vi "test-swerve-drive-kinematics-02.vi"() -> (3 "Test Passed":bool)   [LabVIEW 2019]
uses:
  <vilib>/Rock Robotics/WPI/ThirdParty/JAS_Junk/TrajLib/Trajectory_Library.lvlib
  <vilib>/Rock Robotics/WPI/ThirdParty/JAS_Junk/TrajLib/TypeDef/CHASSIS_SPEEDS.ctl
  <vilib>/Rock Robotics/WPI/ThirdParty/JAS_Junk/TrajLib/TypeDef/ROTATION2D.ctl
  <vilib>/Rock Robotics/WPI/ThirdParty/JAS_Junk/TrajLib/TypeDef/SWERVE_DRIVE_MODULE_STATE.ctl
  <vilib>/Analysis/Matrix/Datatypes/RealMatrix.ctl
  <vilib>/Analysis/Matrix/NI_Matrix.lvlib
  <vilib>/Rock Robotics/WPI/ThirdParty/JAS_Junk/TrajLib/TypeDef/TRANSLATION2D.ctl
  <vilib>/Rock Robotics/WPI/ThirdParty/JAS_Junk/TrajLib/TypeDef/SWERVE_DRIVE_KINEMATICS.ctl
panel:
  out "SWERVE_DRIVE_KINEMATICS":T1 {"SavedModuleStates"."Angle"."SIN" format="%13.4f"; "SavedModuleStates"."Angle"."COS" format="%13.4f"; "SavedModuleStates"."Angle"."VALUE" format="%13.4f"; "PrevCoR"."Y" format="%14.3f"; "PrevCoR"."X" format="%14.3f"; "Modules"."Y" format="%14.3f"; "Modules"."X" format="%14.3f"}
  out "module state":T4={"Speed"=0.0, "Angle"={"VALUE"=0.0, "COS"=1.0, "SIN"=0.0}} {"Angle"."SIN" format="%13.4f"; "Angle"."COS" format="%13.4f"; "Angle"."VALUE" format="%13.4f"}
  out "Chassis Speed":T6 {"vOmega" format="%10.3f"; "vY" format="%10.3f"; "vX" format="%10.3f"}
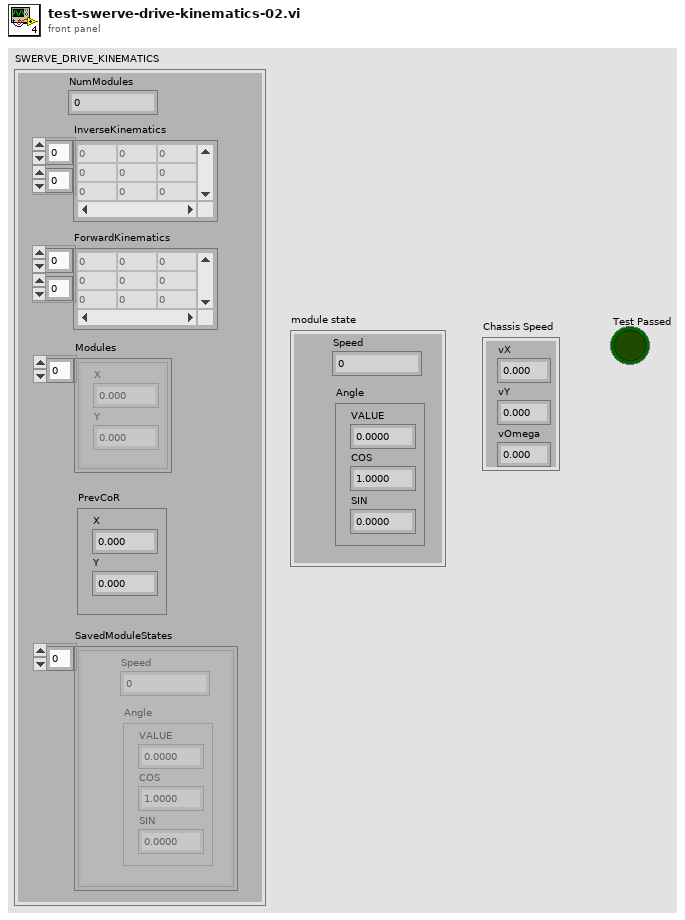
[diagram p1: front panel]
types:
  T1 = typedef "Trajectory_Library.lvlib/SWERVE_DRIVE_KINEMATICS.ctl" = cluster{"NumModules":i32, "InverseKinematics":T2, "ForwardKinematics":T2, "Modules":T3[], "PrevCoR":T3, "SavedModuleStates":T4[]}
  T2 = typedef "NI_Matrix.lvlib/RealMatrix.ctl" = dbl[][]
  T3 = typedef "Trajectory_Library.lvlib/TRANSLATION2D.ctl" = cluster{"X":dbl, "Y":dbl}
  T4 = typedef "Trajectory_Library.lvlib/SWERVE_DRIVE_MODULE_STATE.ctl" = cluster{"Speed":dbl, "Angle":T5}
  T5 = typedef "Trajectory_Library.lvlib/ROTATION2D.ctl" = cluster{"VALUE":dbl, "COS":dbl, "SIN":dbl}
  T6 = typedef "Trajectory_Library.lvlib/CHASSIS_SPEEDS.ctl" = cluster{"vX":dbl, "vY":dbl, "vOmega":dbl}
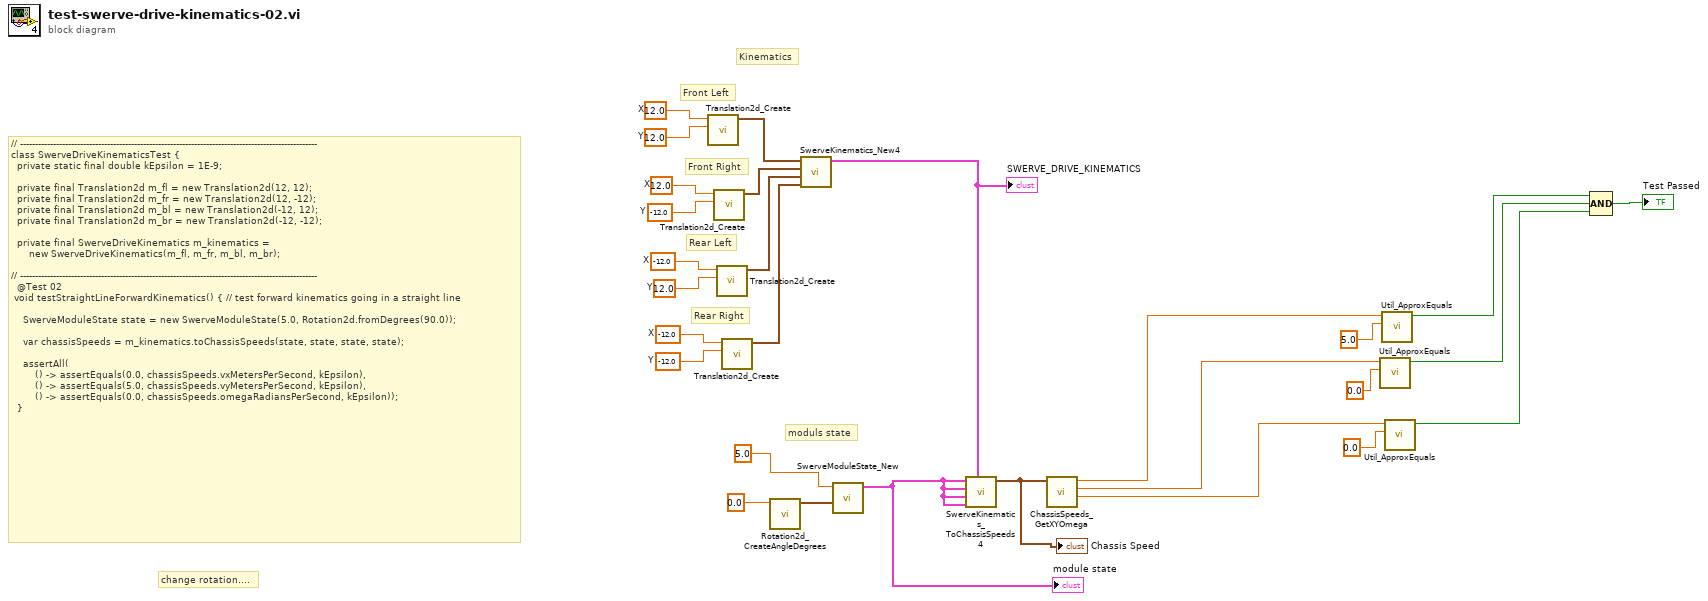
[diagram p0: block diagram]
diagram:
  w24 = -12.0  # X
  w23 = -12.0  # Y
  w22 = -12.0  # X
  w21 = 12.0  # Y
  w20 = 12.0  # X
  w19 = -12.0  # Y
  w18 = 12.0  # X
  w17 = 12.0  # Y
  # "change rotation...."
  # "Kinematics"
  # "Rear Right"
  # "Rear Left"
  # "Front Right"
  # "Front Left"
  # "moduls state"
  # "// ---------------------------------------------------------------------------------------------------\nclass SwerveDriveKinematicsTest {\n  private static final double kEpsilon = 1E-9;\n\n  private final Translation2d m_fl = new Translation2d(12, 12);\n  private final Translation2d m_fr = new Translation2d(12, -12);\n  private final Translation2d m_bl = new Translation2d(-12, 12);\n  private final Translation2d m_br = new Translation2d(-12, -12);\n\n  private final SwerveDriveKinematics m_kinematics =\n      new SwerveDriveKinematics(m_fl, m_fr, m_bl, m_br);\n\n// ---------------------------------------------------------------------------------------------------\n  @Test 02\n void testStraightLineForwardKinematics() { // test forward kinematics going in a straight line\n\n    SwerveModuleState state = new SwerveModuleState(5.0, Rotation2d.fromDegrees(90.0));\n\n    var chassisSpeeds = m_kinematics.toChassisSpeeds(state, state, state, state);\n\n    assertAll(\n        () -> assertEquals(0.0, chassisSpeeds.vxMetersPerSecond, kEpsilon),\n        () -> assertEquals(5.0, chassisSpeeds.vyMetersPerSecond, kEpsilon),\n        () -> assertEquals(0.0, chassisSpeeds.omegaRadiansPerSecond, kEpsilon));\n  }"
  n1 = call <vilib>:"Translation2d_Create.vi"("Y"=w17, "X"=w18) -> ("TRANSLATION"=w25:T3)  [unwired: 9 in]
  n2 = call <vilib>:"Translation2d_Create.vi"("Y"=w19, "X"=w20) -> ("TRANSLATION"=w26:T3)  [unwired: 9 in]
  n3 = call <vilib>:"Translation2d_Create.vi"("Y"=w21, "X"=w22) -> ("TRANSLATION"=w27:T3)  [unwired: 9 in]
  n4 = call <vilib>:"Translation2d_Create.vi"("Y"=w23, "X"=w24) -> ("TRANSLATION"=w28:T3)  [unwired: 9 in]
  n5 = call <vilib>:"Rotation2d_CreateAngleDegrees.vi"("Angle_Degrees"=0.0 ("vY")) -> ("ROTATION"=w7:T5)  [unwired: 10 in]
  n6 = call <vilib>:"SwerveKinematics_New4.vi"("wheel 3"=w28, "wheel 2"=w27, "wheel 1"=w26, "wheel 0"=w25) -> ("SWERVE_DRIVE_KINEMATICS"=w6:T1)  [unwired: 7 in]
  "SWERVE_DRIVE_KINEMATICS" <- w6
  n7 = call <vilib>:"SwerveModuleState_New.vi"("ROTATION"=w7, "Speed"=5.0 ("vX")) -> ("SWERVE_DRIVE_MODULE_STATE"=w5:T4)  [unwired: 9 in]
  "module state" <- w5
  n8 = call <vilib>:"SwerveKinematics_ToChassisSpeeds4.vi"("in SWERVE_DRIVE_KINEMATICS"=w6, "Wheel State 3"=w5, "Wheel State 2"=w5, "Wheel State 1"=w5, "Wheel State 0"=w5) -> ("Chassis Speed"=w1:T6)  [unwired: 6 in]
  "Chassis Speed" <- w1
  n9 = call <vilib>:"ChassisSpeeds_GetXYOmega.vi"("CHASSIS"=w1) -> ("vAngular"=w2:dbl, "vY"=w3:dbl, "vX"=w4:dbl)  [unwired: 8 in]
  n10 = call <vilib>:"Util_ApproxEquals.vi"("Value 2"=0.0, "Value 1"=w3) -> ("ApproxEquals"=w12:bool)  [unwired: 9 in]
  n11 = call <vilib>:"Util_ApproxEquals.vi"("Value 2"=5.0, "Value 1"=w4) -> ("ApproxEquals"=w13:bool)  [unwired: 9 in]
  n12 = call <vilib>:"Util_ApproxEquals.vi"("Value 2"=0.0, "Value 1"=w2) -> ("ApproxEquals"=w11:bool)  [unwired: 9 in]
  n13 = Compound Arithmetic op=AND(w13, w12, w11) -> (→"Test Passed":bool)
